vi "SECoP_dataGetBool.vi"(7 "Position":u32, 8 "error in (no error)":errorcluster, 9 "Index":u32, 10 "SECoP_dataPtr":T1 {"ptr64" format="%.0x"; "ptr32" format="%.0x"}, 11 "DLL path (in)":T2) -> (0 "error out":errorcluster, 2 "Boolean":bool, 3 "DLL path (out)":T2)   [LabVIEW 2023, in "SECoP.lvlib"]
doc: "Call <b>\"SECoP_dataGetBool.vi\"</b> to access the boolean value (SECoP_dataPtr).\n\n<b>DLL path</b> input and output of cluster from \"SECoP-Initialize.vi\"\n<b>SECoP_dataPtr</b> data to access\n<b>Position</b> points to a virtual flattened entry of the data type\n<b>Index</b> zero based index into array type or 0 for single type\n<b>Value</b> boolean value (True only, if value is non-zero)"
uses:
  SECoP.lvlib
  SECoP-libraries.ctl
  SECoP-data.ctl
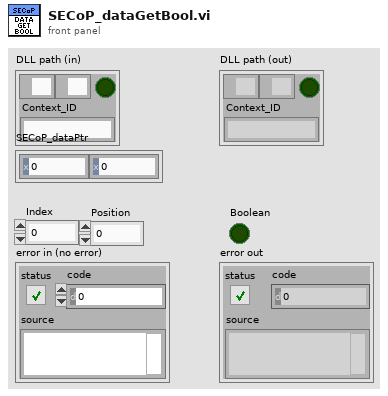
[diagram p1: front panel]
types:
  T1 = typedef "SECoP.lvlib/SECoP-data.ctl" = cluster{"ptr32":u32, "ptr64":u64}
  T2 = typedef "SECoP.lvlib/SECoP-libraries.ctl" = cluster{"serverDLL":path, "variantDLL":path, "cleanup_mode":bool, "Context_ID":string}
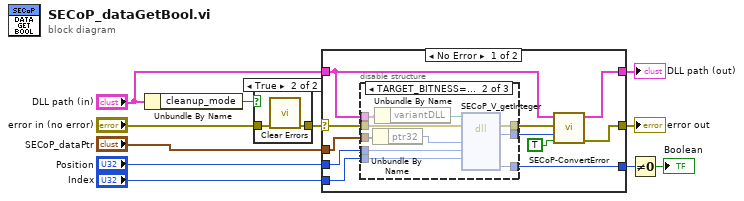
[diagram p0: block diagram]
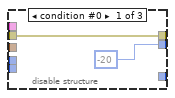
[diagram p3: hidden frame]
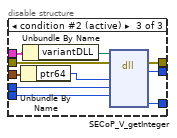
[diagram p4: hidden frame]
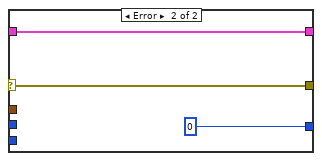
[diagram p5: hidden frame]
diagram:
  n1 = Unbundle By Name("DLL path (in)") -> ("cleanup_mode"=w8:bool)
  n2 = case shown="True" w8 {
    tunnel: "error in (no error)" -> [w12 w14]
    tunnel: [w12 w13] -> w6
    frame False {
    }
    frame True {
      n3 = call <vilib>:"Clear Errors.vi"("error in (no error)"=w14) -> ("error out"=w13:errorcluster)  [unwired: 5 in, 1 out]
    }
  }
  n4 = case shown="No Error" w6 {
    selector: w6 -> [w23 w49]
    tunnel: "DLL path (in)" -> [w15 w50]
    tunnel: [w24 w50] -> w10
    tunnel: [w25 w49] -> w9
    tunnel: "Position" -> [w19 _]
    tunnel: "Index" -> [w18 _]
    tunnel: [w17 i64 0 ("Value")] -> w3
    tunnel: "SECoP_dataPtr" -> [w16 _]
    frame No Error {
      n5 = disable-structure shown="TARGET_BITNESS==32" {
        disable-tunnel: w23 -> [w27 w37 w47]
        disable-tunnel: w15 -> [_ w36 w46]
        disable-tunnel: [w27 w35 w45] -> w22
        disable-tunnel: [-20 w34 w44] -> w21
        disable-tunnel: w19 -> [_ w33 w43]
        disable-tunnel: w18 -> [_ w32 w42]
        disable-tunnel: [_ w31 w41] -> w17
        disable-tunnel: w16 -> [_ w30 w40]
        frame condition #0 {
        }
        frame condition #1 {
          n6 = Unbundle By Name(w30) -> ("ptr32"=w29:u32)
          n7 = Unbundle By Name(w36) -> ("variantDLL"=w28:path)
          n8 = dll-call lib="Z:/Praktische_Aufgaben/SECoP-LabVIEW2015/32bit/SECoP32.dll" fn="SECoP_V_getInteger"(path in=w28, error in=w37, "Data"=w29, "Position"=w33, "Index"=w32) -> (error out=w35:errorcluster, "return type"=w34:i32, "Value"=w31:i64)  [unwired: 5 in, 1 out]
        }
        frame condition #2 (active) {
          n9 = Unbundle By Name(w40) -> ("ptr64"=w39:u64)
          n10 = Unbundle By Name(w46) -> ("variantDLL"=w38:path)
          n11 = dll-call lib="Z:/Praktische_Aufgaben/SECoP-LabVIEW2015/32bit/SECoP32.dll" fn="SECoP_V_getInteger"(path in=w38, error in=w47, "Data"=w39, "Position"=w43, "Index"=w42) -> (error out=w45:errorcluster, "return type"=w44:i32, "Value"=w41:i64)  [unwired: 5 in, 1 out]
        }
      }
      n12 = call "SECoP-ConvertError.vi"("return is boolean"=TRUE, "return code"=w21, "error in (no error)"=w22, "DLL path (in)"=w15) -> ("error out"=w25:errorcluster, "DLL path (out)"=w24:T2)  [unwired: 6 in]
    }
    frame Error {
    }
  }
  "DLL path (out)" <- w10
  "error out" <- w9
  n13 = Not Equal To 0?(x=w3) -> (x != 0?=→"Boolean":bool)
